vi "String2ArrayInt.vi"(3 "R_message 1":string) -> (0 "Value_ind0":i32, 1 "ArrayInt":i32[](array[numeric]))   [LabVIEW 2022 SP3]
panel:
  out "subarray":u8[](array[numeric]) format="%x"
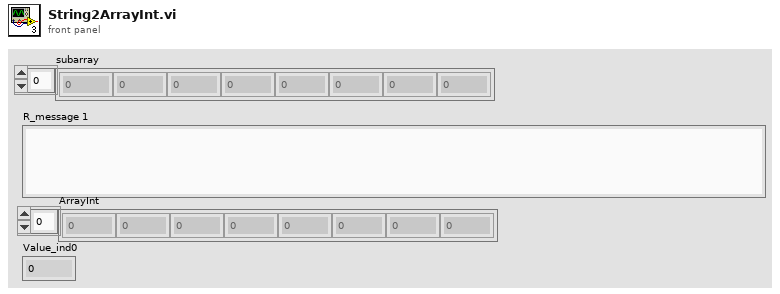
[diagram p1: front panel]
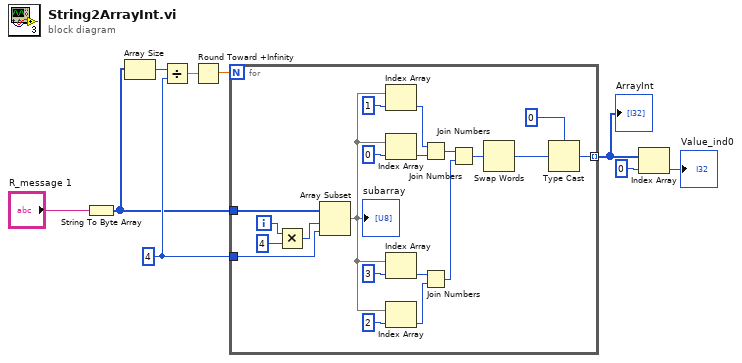
[diagram p0: block diagram]
diagram:
  w7 = 4 ("length")
  n1 = String To Byte Array(string="R_message 1") -> (unsigned byte array=w4:u8[])
  n2 = Array Size(array=w4) -> (size(s)=w8:i32)
  n3 = Divide(x=w8, y=w7) -> (x/y=w6:dbl)
  n4 = Round Toward +Infinity(x=w6) -> (ceil(x): smallest int >= x=w5:dbl)
  n5 = for {
    N: w5 -> [_]
    tunnel: w4 -> [w29]
    tunnel: w7 -> [w28]
    tunnel: [w27] -> w3 mode=indexing
    i -> [w13]
    n6 = Multiply(x=w13, y=4) -> (x*y=w11:i32)
    n7 = Array Subset(array=w29, index=w11, length=w28) -> (w18:u8[])
    "subarray" <- w18
    n8 = Index Array(array=w18, index=1) -> (element=w20:u8)
    n9 = Index Array(array=w18, index=0) -> (element=w19:u8)
    n10 = Index Array(array=w18, index=3) -> (element=w17:u8)
    n11 = Index Array(array=w18, index=2) -> (element=w16:u8)
    n12 = Join Numbers(hi=w20, lo=w19) -> ((hi.lo)=w21:u16)
    n13 = Join Numbers(hi=w17, lo=w16) -> ((hi.lo)=w22:u16)
    n14 = Join Numbers(hi=w21, lo=w22) -> ((hi.lo)=w15:u32)
    n15 = Swap Words(1:w15) -> (0:w14:u32)
    n16 = Type Cast(type=0, x=w14) -> (*(type *) &x=w27:i32)
  }
  "ArrayInt" <- w3
  n17 = Index Array(array=w3, index=0) -> (element=→"Value_ind0":i32)
